vi "host_main.vi"() -> ()   [LabVIEW 2020]
uses:
  control/host_data.ctl
  Real_Time/control/logging_data.ctl
  Real_Time/control/system_monitoring_data.ctl
  sub_vi/PlotGraph.llb/GraphPlot.lvlib
panel:
  in  "Arm_down_sig":u8
  in  "Bucket_down_sig":u8
  in  "Boom_down_sig":u8
  out "z_aixs_position(mm)":dbl format="%.1f"
  in  "Bucket_up_sig":u8
  in  "Arm_up_sig":u8
  in  "Boom_up_sig":u8
  out "Bucket_vale":dbl format="%.1f"
  in  "logging_enable":bool
  out "Arm_vale":dbl format="%.1f"
  out "Boom_valve":dbl format="%.1f"
  out "x_aixs_position(mm)":dbl format="%.1f"
  out "logging_state":bool
  out "Bucket":dbl format="%.1f"
  out "Arm":dbl format="%.1f"
  out "Boom":dbl format="%.1f"
  out "rt_system_elapse_time":string
  out "rt_system_absolute_time":string
  out "rt_system_temp":dbl
  out "rt_system_load":dbl
  out "valve_signal_graph":cluster{dbl[], dbl[]}[](graph)
  out "AngualrPositionGraph":cluster{dbl[], dbl[]}[](graph)
  in  "stop":bool
  in  "GraphLength(sec)":dbl=60.0
  out "angle_graph":cluster{dbl[], dbl[]}[](graph)
  # "Manual Control"
  # "System Status"
  # "Monitoring Stop"
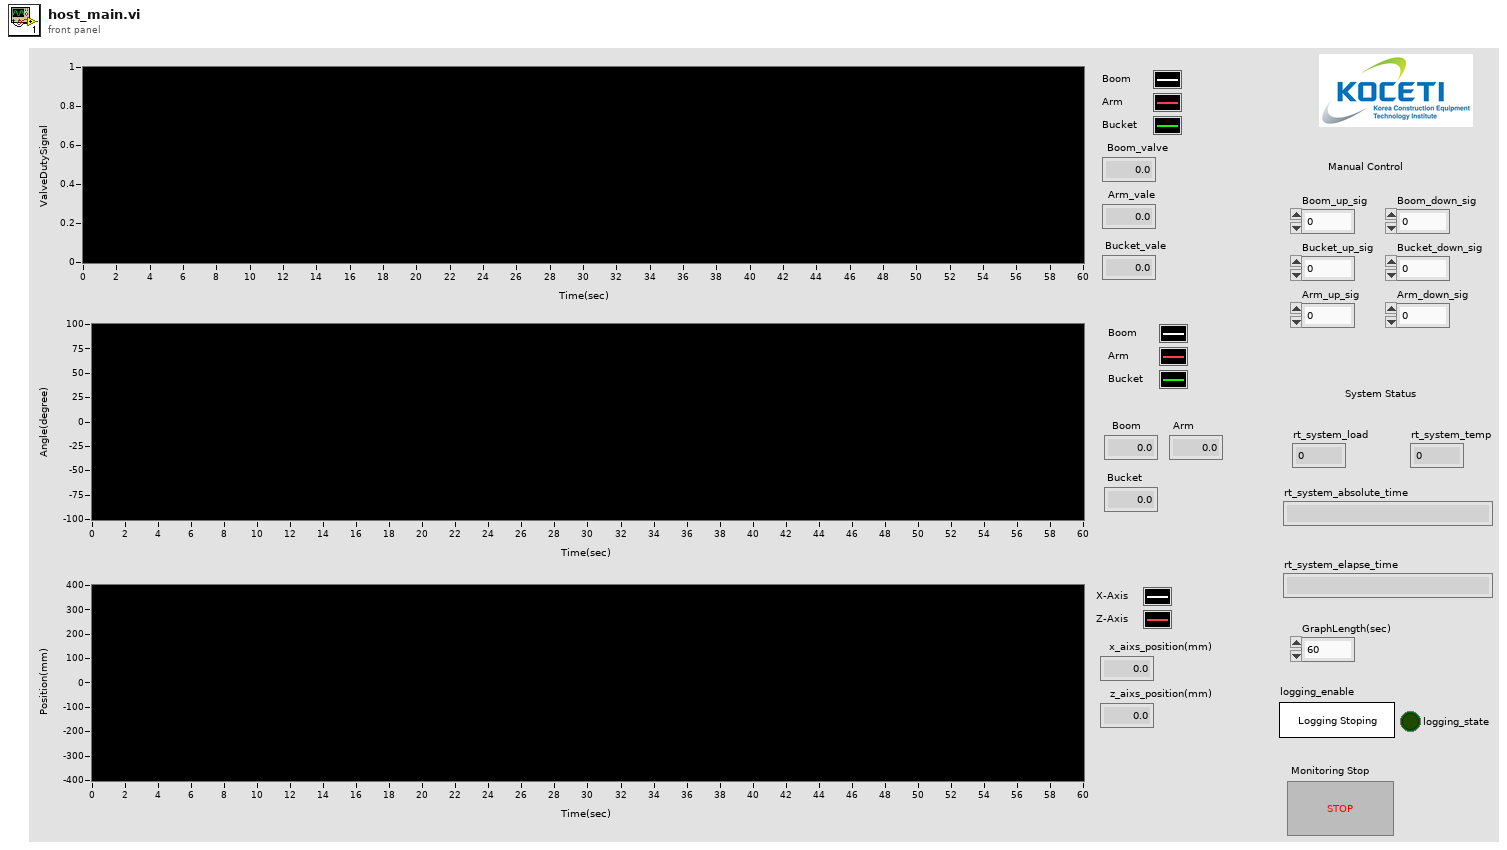
[diagram p1: front panel]
types:
  T1 = typedef "host_data.ctl" = cluster{"logging_enable":bool, "boom_up_signal":u8, "boom_down_signal":u8, "arm_up_signal":u8, "arm_down_signal":u8, "bucket_up_signal":u8, "bucket_down_signal":u8}
  T2 = typedef "system_monitoring_data.ctl" = cluster{"logging_state":bool, "rt_system_load":dbl, "rt_system_temp":dbl, "rt_system_absolute_time":string, "rt_system_elapse_time":string}
  T3 = typedef "logging_data.ctl" = cluster{"time(sec)":dbl, "boom_valve_pwm":dbl, "arm_valve_pwm":dbl, "bucket_valve_pwm":dbl, "boom_angle":dbl, "arm_angle":dbl, "bucket_angle":dbl, "x_aixs_position":i32, "z_aixs_position":i32}
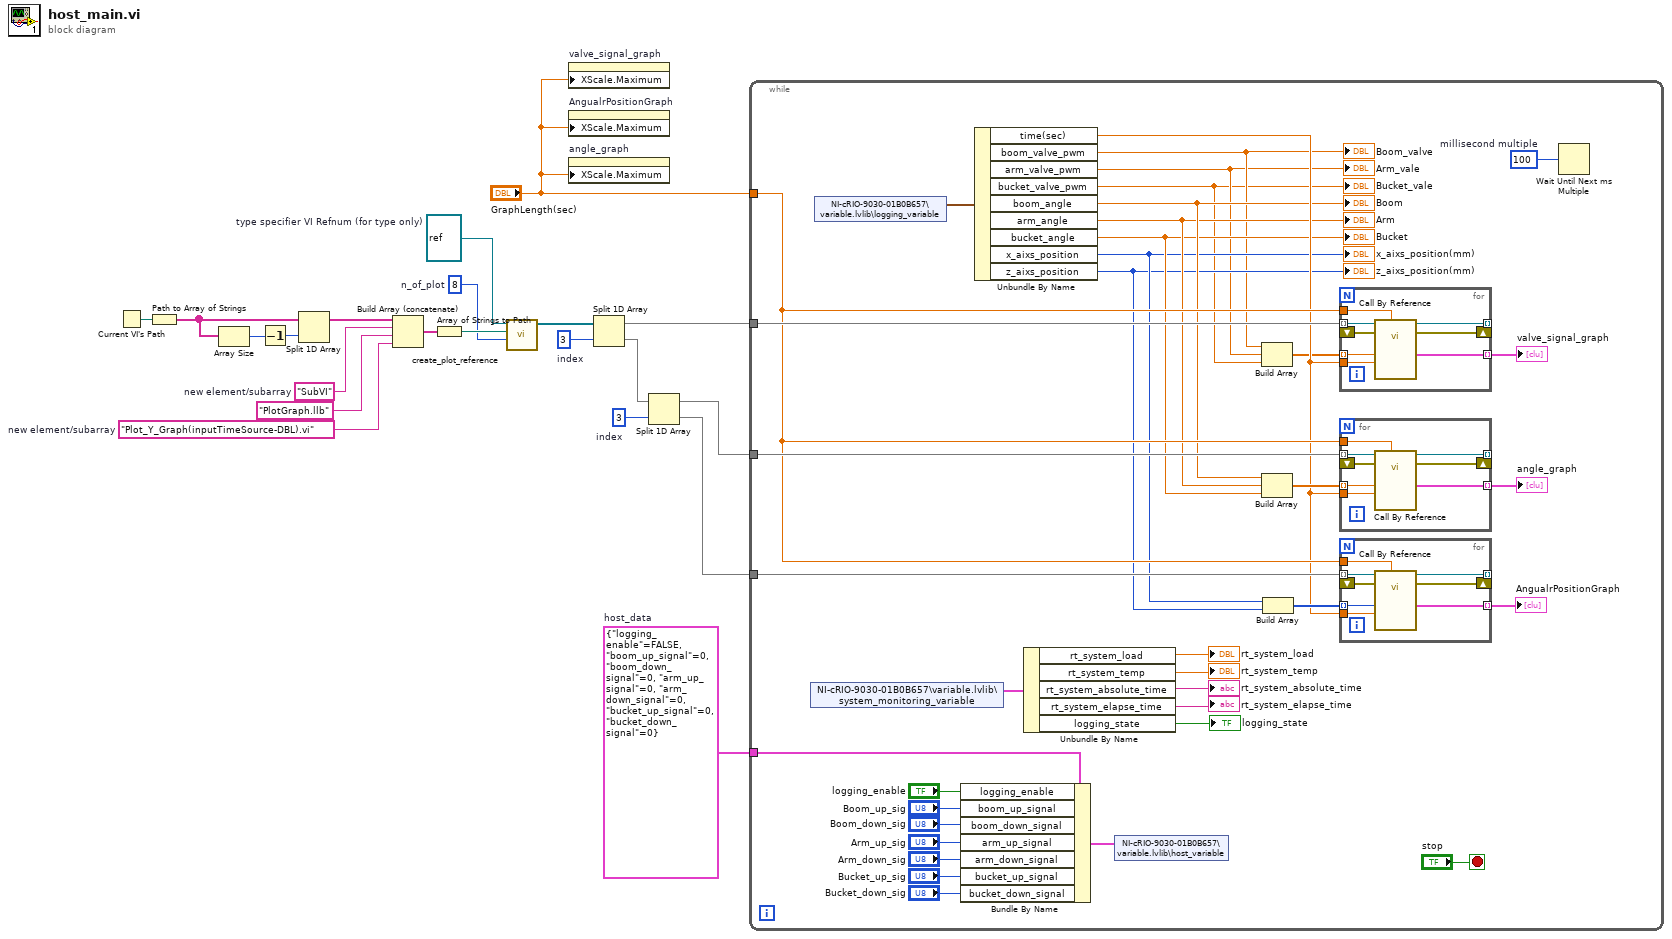
[diagram p0: block diagram]
diagram:
  w1 = T1 {"logging_enable"=FALSE, "boom_up_signal"=0, "boom_down_signal"=0, "arm_up_signal"=0, "arm_down_signal"=0, "bucket_up_signal"=0, "bucket_down_signal"=0}  # host_data
  w2 = 8  # n_of_plot
  w3 = 3  # index
  w8 = 3  # index
  w15 = "Plot_Y_Graph(inputTimeSource-DBL).vi"  # new element/subarray
  w12 = "SubVI"  # new element/subarray
  w14 = refnum<vi> refnum  # type specifier VI Refnum (for type only)
  n1 = Current VI's Path() -> (path=w21:path)
  n2 = Path to Array of Strings(0:w21) -> (2:w20:string[])  [unwired: 1 out]
  n3 = Array Size(array=w20) -> (size(s)=w19:i32)
  n4 = Decrement(x=w19) -> (x-1=w18:i32)
  n5 = Split 1D Array(array=w20, index=w18) -> (first subarray=w17:string[])  [unwired: 1 out]
  n6 = Build Array (concatenate) "Build Array"(w17, w12, "PlotGraph.llb", w15) -> (w16:string[])
  n7 = Array of Strings to Path(0:w16) -> (2:w13:path)  [unwired: 1 in]
  n8 = call "create_plot_reference.vi"("n_of_plot"=w2, "path_of_plot"=w13, "plot_prototype"=w14) -> ("ref_of_plot"=w9:refnum<vi>[])  [unwired: 7 in, 1 out]
  n9 = property on="valve_signal_graph" class="XYGraph (strict)"("XScale.Maximum"="GraphLength(sec)") -> ()  [unwired: 2 in, 2 out]
  n10 = property on="AngualrPositionGraph" class="XYGraph (strict)"("XScale.Maximum"="GraphLength(sec)") -> ()  [unwired: 2 in, 2 out]
  n11 = property on="angle_graph" class="XYGraph (strict)"("XScale.Maximum"="GraphLength(sec)") -> ()  [unwired: 2 in, 2 out]
  n12 = Split 1D Array(array=w9, index=w8) -> (first subarray=w7:refnum<vi>[], second subarray=w6:refnum<vi>[])
  n13 = Split 1D Array(array=w6, index=w3) -> (first subarray=w5:refnum<vi>[], second subarray=w4:refnum<vi>[])
  n14 = while {
    tunnel: w7 -> [w55]
    tunnel: "GraphLength(sec)" -> [w50]
    tunnel: w5 -> [w53]
    tunnel: w4 -> [w51]
    tunnel: w1 -> [w44]
    stop <- "stop" stop-if-true
    w56 = u32 100  # millisecond multiple
    n15 = shared-variable "NI-cRIO-9030-01B0B657\\variable.lvlib\\system_monitoring_variable"() -> (w49:T2)  [unwired: 1 in, 1 out]
    n16 = shared-variable "NI-cRIO-9030-01B0B657\\variable.lvlib\\logging_variable"() -> (w58:T3)  [unwired: 1 in, 1 out]
    n17 = Bundle By Name(cluster=w44, "logging_enable"="logging_enable", "boom_up_signal"="Boom_up_sig", "boom_down_signal"="Boom_down_sig", "arm_up_signal"="Arm_up_sig", "arm_down_signal"="Arm_down_sig", "bucket_up_signal"="Bucket_up_sig", "bucket_down_signal"="Bucket_down_sig") -> (w28:T1)
    n18 = Unbundle By Name(w58) -> ("time(sec)"=w43:dbl, "boom_valve_pwm"=w32:dbl, "arm_valve_pwm"=w31:dbl, "bucket_valve_pwm"=w30:dbl, "boom_angle"=w37:dbl, "arm_angle"=w36:dbl, "bucket_angle"=w35:dbl, "x_aixs_position"=w34:i32, "z_aixs_position"=w33:i32)
    "Boom" <- w37
    "Arm" <- w36
    "Bucket" <- w35
    "x_aixs_position(mm)" <- w34
    "Boom_valve" <- w32
    "Arm_vale" <- w31
    "Bucket_vale" <- w30
    "z_aixs_position(mm)" <- w33
    n19 = Unbundle By Name(w49) -> ("rt_system_load"=→"rt_system_load":dbl, "rt_system_temp"=→"rt_system_temp":dbl, "rt_system_absolute_time"=→"rt_system_absolute_time":string, "rt_system_elapse_time"=→"rt_system_elapse_time":string, "logging_state"=→"logging_state":bool)
    n20 = shared-variable "NI-cRIO-9030-01B0B657\\variable.lvlib\\host_variable"(w28) -> ()  [unwired: 1 in, 1 out]
    n21 = Build Array(w32, w31, w30) -> (w29:dbl[])
    n22 = Build Array(w37, w36, w35) -> (w54:dbl[])
    n23 = Build Array(w34, w33) -> (w52:i32[])
    n24 = for {
      tunnel: w55 -> [w76] mode=indexing
      tunnel: [w82] -> w39 mode=indexing
      tunnel: w29 -> [w81] mode=indexing
      tunnel: w50 -> [w77]
      shift-right: [w80] -> _
      shift-left: _ -> [w79]
      tunnel: [w78] -> _ mode=indexing
      tunnel: w43 -> [w75]
      n25 = call-by-ref "Call By Reference"(reference=w76, error in=w79, "GraphLength(sec)"=w77, "TimeSource"=w75, "DataInput(Y-Value)"=w81) -> (reference out=w78:refnum<vi>, error out=w80:errorcluster, "output_plot"=w82:cluster{dbl[], dbl[]})  [unwired: 8 in]
    }
    "valve_signal_graph" <- w39
    n26 = for {
      tunnel: w53 -> [w68] mode=indexing
      tunnel: [w74] -> w38 mode=indexing
      tunnel: w54 -> [w73] mode=indexing
      tunnel: w50 -> [w69]
      shift-right: [w72] -> _
      shift-left: _ -> [w71]
      tunnel: [w70] -> _ mode=indexing
      tunnel: w43 -> [w67]
      n27 = call-by-ref "Call By Reference"(reference=w68, error in=w71, "GraphLength(sec)"=w69, "TimeSource"=w67, "DataInput(Y-Value)"=w73) -> (reference out=w70:refnum<vi>, error out=w72:errorcluster, "output_plot"=w74:cluster{dbl[], dbl[]})  [unwired: 8 in]
    }
    "angle_graph" <- w38
    n28 = for {
      tunnel: w51 -> [w60] mode=indexing
      tunnel: [w66] -> w27 mode=indexing
      tunnel: w52 -> [w65] mode=indexing
      tunnel: w50 -> [w61]
      shift-right: [w64] -> _
      shift-left: _ -> [w63]
      tunnel: [w62] -> _ mode=indexing
      tunnel: w43 -> [w59]
      n29 = call-by-ref "Call By Reference"(reference=w60, error in=w63, "GraphLength(sec)"=w61, "TimeSource"=w59, "DataInput(Y-Value)"=w65) -> (reference out=w62:refnum<vi>, error out=w64:errorcluster, "output_plot"=w66:cluster{dbl[], dbl[]})  [unwired: 8 in]
    }
    "AngualrPositionGraph" <- w27
    n30 = Wait Until Next ms Multiple(millisecond multiple=w56) -> ()  [unwired: 1 out]
  }
